vi "VI-Get XControl State Cluster.vi"(0 "XControlLibrary in":refnum<vi>, 11 "error in (no error)":errorcluster) -> (4 "XControlLibrary out":refnum<vi>, 6 "VI ref":refnum<vi>, 8 "State cluster":refnum<vi>, 15 "error out":errorcluster)   [LabVIEW 2015]
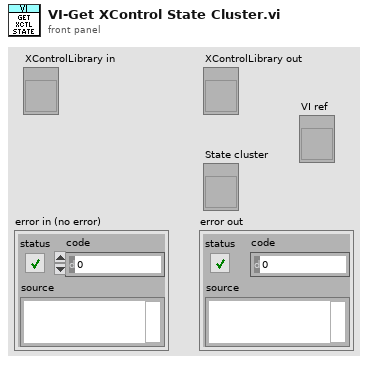
[diagram p1: front panel]
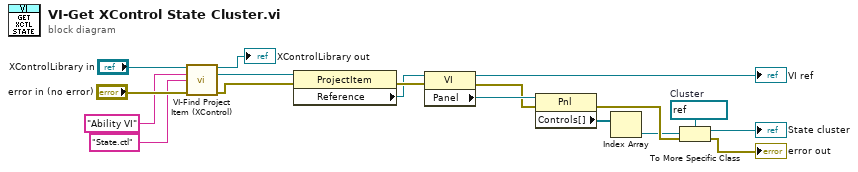
[diagram p0: block diagram]
diagram:
  w13 = refnum<vi> refnum  # Cluster
  n1 = call "VI-Find Project Item (XControl).vi"("XCtlLib Refnum"="XControlLibrary in", "Type"="Ability VI", "Name"="State.ctl", "error in (no error)"="error in (no error)") -> ("reference out"=→"XControlLibrary out":refnum<vi>, "ProjectItem"=w8:refnum<vi>, "error out"=w18:errorcluster)  [unwired: 9 in]
  n2 = property class="ProjectItem"(reference=w8, error in=w18) -> (error out=w16:errorcluster, "Reference"=w9:refnum<vi>)  [unwired: 1 out]
  n3 = property class="VI"(reference=w9, error in=w16) -> (reference out=→"VI ref":refnum<vi>, error out=w4:errorcluster, "Panel"=w10:refnum<vi>)
  n4 = property class="Pnl"(reference=w10, error in=w4) -> (error out=w17:errorcluster, "Controls[]"=w11:refnum<vi>[])  [unwired: 1 out]
  n5 = Index Array(array=w11) -> (element=w12:refnum<vi>)  [unwired: 1 in]
  n6 = To More Specific Class(target class=w13, reference=w12, error in=w17) -> (specific class reference=→"State cluster":refnum<vi>, error out=→"error out":errorcluster)
